vi "Read MongoDB.Database.vi"(8 "error in (no error)":errorcluster, 11 "MongoDB.Database in":refnum<class "MongoDB.Database.lvclass">) -> (0 "error out":errorcluster, 2 "MongoDB.Database":refnum<k24>, 3 "MongoDB.Database out":refnum<class "MongoDB.Database.lvclass">)   [LabVIEW 2014, in "MongoDB.Database.lvclass"]
uses:
  MongoDB.Database.lvclass
  C:/MongoData/Drivers/mongo-csharp-driver-2.0.0-beta4/mongo-csharp-driver-2.0.0-beta4/src/MongoDB.Driver.Legacy/bin/Release/MongoDB.Driver.Legacy.dll
  MongoData/Drivers/mongo-csharp-driver-2.0.0-beta4/mongo-csharp-driver-2.0.0-beta4/src/MongoDB.Driver.Legacy/bin/Release/MongoDB.Driver.Legacy.dll
  MongoDB.Database.lvclass/MongoDB.Database.ctl
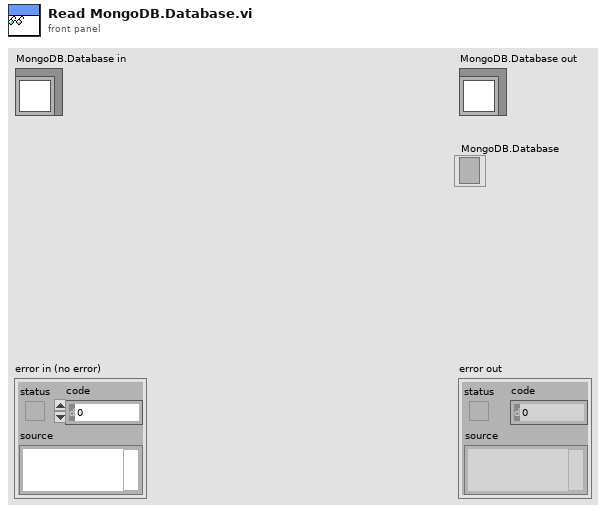
[diagram p1: front panel]
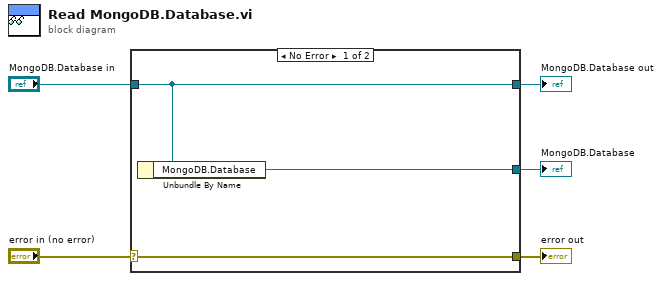
[diagram p0: block diagram]
diagram:
  n1 = case shown="No Error" "error in (no error)" {
    selector: "error in (no error)" -> [w8 w9]
    tunnel: [w8 w9] -> w4
    tunnel: [w7 w10] -> w2
    tunnel: "MongoDB.Database in" -> [w7 w10]
    tunnel: [w6 _] -> w1
    frame No Error {
      n2 = Unbundle By Name(w7) -> ("MongoDB.Database"=w6:refnum<k24>)
    }
    frame Error {
    }
  }
  "error out" <- w4
  "MongoDB.Database out" <- w2
  "MongoDB.Database" <- w1
